vi "APS point table move3.vi"(7 "EndIndex":i32, 8 "error in (no error)":errorcluster caption="错误输入（无错误）", 9 "StartIndex":i32, 10 "Axis_ID_Array":i32, 11 "Dimension":i32) -> (0 "error out":errorcluster caption="错误输出", 2 "Axis_ID_Array out":i32, 3 "function return":i32)   [LabVIEW 2011, in "APS168.lvlib"]
doc: "I32 FNTYPE APS_point_table_move3( I32 Dimension, I32 *Axis_ID_Array, I32 StartIndex, I32 EndIndex );"
uses:
  APS168.lvlib
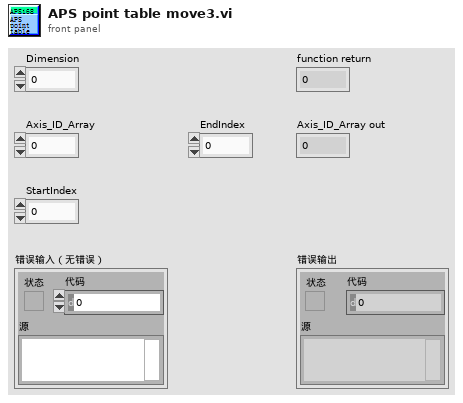
[diagram p1: front panel]
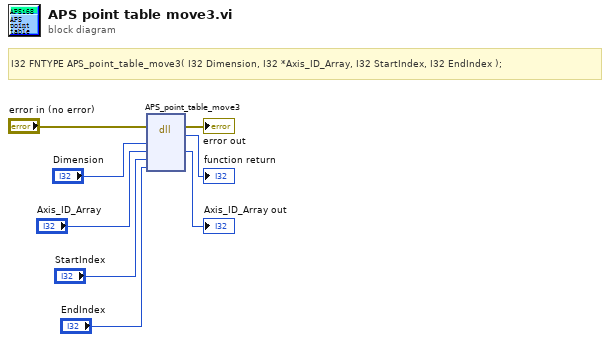
[diagram p0: block diagram]
diagram:
  # "I32 FNTYPE APS_point_table_move3( I32 Dimension, I32 *Axis_ID_Array, I32 StartIndex, I32 EndIndex );"
  n1 = dll-call lib="PTH1Labs E软件ADLINK 204CAPS_1_7_1_LIB line 连续运动204APS168.*" fn="APS_point_table_move3"(error in="error in (no error)", "Dimension"="Dimension", "Axis_ID_Array"="Axis_ID_Array", "StartIndex"="StartIndex", "EndIndex"="EndIndex") -> (error out=→"error out":errorcluster, →"function return":i32, "Axis_ID_Array"=→"Axis_ID_Array out":i32)  [unwired: 5 in, 1 out]
